vi "dfd_Direct IIR I Normalization.vi"(7 "scale type":T1, 9 "coefficients b":dbl[](array[numeric]) format="%.2f", 10 "coefficients a":dbl[](array[numeric]) format="%.2f", 11 "x":dbl[](array[numeric])) -> (2 "norm":dbl[](array[numeric]) format="%.2f", 3 "y":dbl[](array[numeric]))   [LabVIEW 2017, in "NI_DigFilter_FXP.lvlib"]
uses:
  <vilib>/addons/Digital Filter Design/NI_DigFilter_FXP.lvlib
  <vilib>/addons/Digital Filter Design/_Objects.llb/DFD Coef Norm Type.ctl
  <vilib>/addons/Digital Filter Design/NI_DigFilterLicensed.lvlib
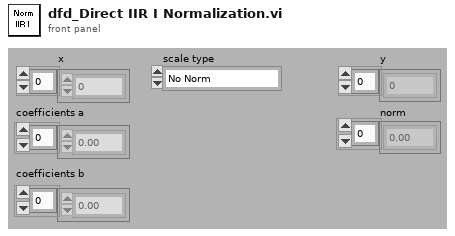
[diagram p1: front panel]
types:
  T1 = typedef "NI_DigFilterLicensed.lvlib/DFD Coef Norm Type.ctl" = enum16{"No Norm", "Time Domain 1-Norm", "Time Domain 2-Norm", "Time Domain Inf-Norm"}
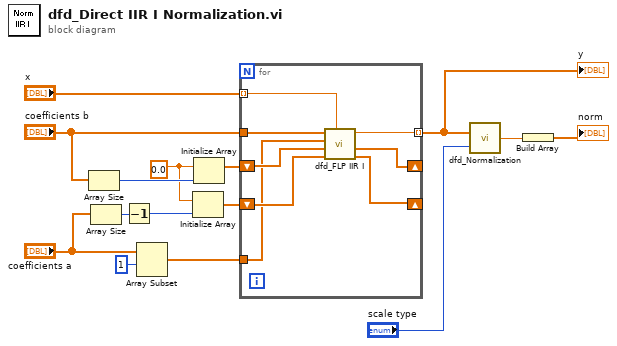
[diagram p0: block diagram]
diagram:
  w3 = 0.0 ("element")
  n1 = Array Size(array="coefficients b") -> (size(s)=w4:i32)
  n2 = Array Size(array="coefficients a") -> (size(s)=w11:i32)
  n3 = Decrement(x=w11) -> (x-1=w5:i32)
  n4 = Array Subset(array="coefficients a", index=1) -> (w9:dbl[])  [unwired: 1 in]
  n5 = Initialize Array(w3, w5) -> (w8:dbl[])
  n6 = Initialize Array(w3, w4) -> (w15:dbl[])
  n7 = for {
    shift-right: [w20] -> _
    shift-left: w15 -> [w22]
    tunnel: [w18] -> w1 mode=indexing
    shift-right: [w19] -> _
    shift-left: w8 -> [w21]
    tunnel: "coefficients b" -> [w23]
    tunnel: w9 -> [w17]
    tunnel: "x" -> [w16] mode=indexing
    (unwired) 0.0 ("element")
    n8 = call <vilib>:"dfd_FLP IIR I.vi"("x"=w16, "y states in"=w21, "x states in"=w22, "coefficients a"=w17, "coefficents b"=w23) -> ("y states out"=w19:dbl[], "x states out"=w20:dbl[], "y"=w18:dbl)  [unwired: 4 out]
  }
  "y" <- w1
  n9 = call <vilib>:"dfd_Normalization.vi"("scale type"="scale type", "h(n)"=w1) -> ("norm"=w13:dbl)
  n10 = Build Array(w13) -> (→"norm":dbl[])
